vi "Constants.vi"() -> ()   [LabVIEW 2014, in "VeriStand Steps Version Mutation.lvlib"]
uses:
  VeriStand Steps Version Mutation.lvlib
panel:
  in  "TypePalette File Name":string="NI_VeriStandTypes.ini"
  in  "CSharp Project File Name":string="VeristandSteps.csproj"
  in  "CSharp Project Folder Name":string="OpenWorkspaceDialog"
  in  "CSharp Solution Folder Name":string="VeristandStepsInstaller"
  in  "TypePalette Folder Name":string="TypePalette INI File"
  in  "LV Code Folder Name":string="LabVIEW Code"
  in  "CSharp Code Folder Name":string="C# Code"
  in  "VeriStand Silent Start Project Name":string="SilentVS.lvproj"
  in  "VeriStand Silent Start Project Folder Name":string="VeriStand Silent Start"
  in  "TS VS Logger Project Name":string="TS VS Logger.lvproj"
  in  "TS VS Logger Project Folder Name":string="TS VS Logger"
  in  "Set Channels Project Name":string="Set Channels.lvproj"
  in  "Set Channels Project Folder Name":string="Set Channels"
  in  "RT Sequence Project Name":string="RTSequenceVIs.lvproj"
  in  "RT Sequence Project Folder Name":string="RT Sequence"
  in  "MiscHelperVIs Project Name":string="MiscHelperVIs.lvproj"
  in  "MiscHelperVIs Project Folder Name":string="Misc"
  # "LabVIEW Constants"
  # "dotNET Constants"
  # "TestStand Constants"
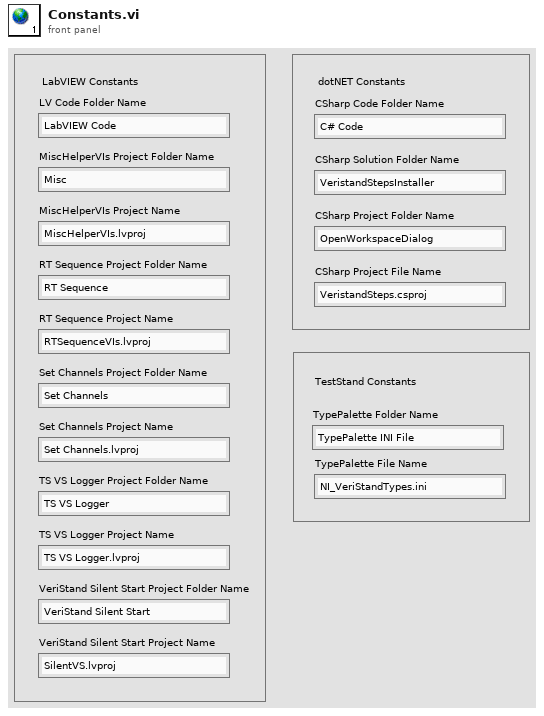
[diagram p1: front panel]
diagram:
